vi "timer_correct_rollover.vi"(9 "Reset":bool, 10 "Loop Rate(uSec)":u64) -> (0 "Actual Loop Rate(uSec)":u64, 1 "Late? (Latched)":bool, 2 "Tick Count(uSec)":u64)   [LabVIEW 2014]
doc: "This VI will monitor the rate of a loop on FPGA. It calculates the number of ticks that have passed since the last call and compares it with the desired count. If more ticks have passed than desired, the Late? Boolean latches to TRUE until reset.\n\n<B>Inputs:</B>\n<B>Count(Ticks)</B> - The desired number of ticks since the last call.\n<B>Reset</B> - Resets the Late? Boolean.\n\n<B>Outputs:</B>\n<B>Tick Count (Ticks)</B> - Returns the value of the free running tick counter.\n<B>Late? (Latched)</B> - Indicates if more FPGA Ticks have passed than the specified number. This Boolean value is latched until reset.\n<B>Actual Loop Rate (Ticks)</B> - The number of ticks that have passed since the last call."
uses:
  Instance           2 36Saved   Monitor Loop Rate - Latching .vi
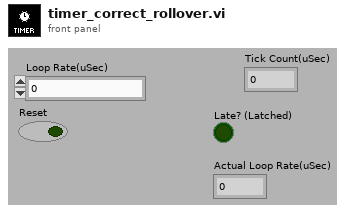
[diagram p1: front panel]
types:
  T1 = cluster{bool, "code":i32, "error_message":string}
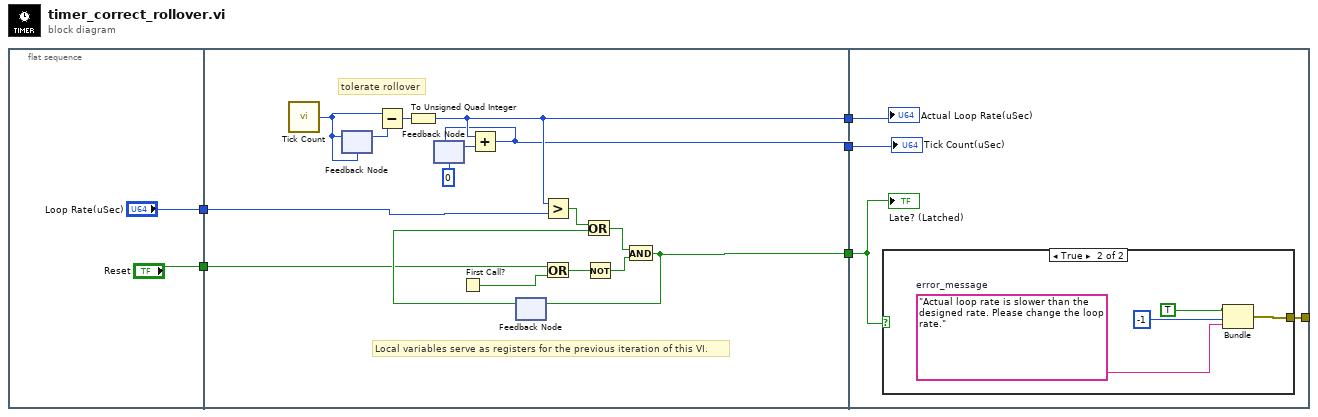
[diagram p0: block diagram]
diagram:
  n1 = flat-sequence {
    tunnel: ["Loop Rate(uSec)"] -> w4
    tunnel: ["Reset"] -> w3
    tunnel: [w12] -> w5
    tunnel: w4 -> [w11]
    tunnel: w3 -> [w10]
    tunnel: [w9] -> w2
    tunnel: [w8] -> w1
    tunnel: w5 -> [w25]
    tunnel: w2 -> [w27]
    tunnel: w1 -> [w26]
    tunnel: [w24] -> _
    frame #0 {
    }
    frame #1 {
      # "tolerate rollover"
      # "Local variables serve as registers for the previous iteration of this VI."
      n2 = call "Tick Count"() -> ("Tick Count(uSec)"=w13:u32)
      n3 = feedback #1(w13) -> (w17:u32)
      n4 = feedback-in #1(w13) -> ()
      n5 = Subtract(x=w13, y=w17) -> (x-y=w14:u32)
      n6 = To Unsigned Quad Integer(1:w14) -> (0:w9:u64)
      n7 = feedback #2(u64 0 ("Tick Count(uSec)")) -> (w15:u64)
      n8 = First Call?() -> (First Call?: T/F=w22:bool)
      n9 = Add(x=w9, y=w15) -> (x+y=w8:u64)
      n10 = feedback-in #2(w8) -> ()
      n11 = feedback #3() -> (w18:bool)  [unwired: 1 in]
      n12 = Greater?(x=w9, y=w11) -> (0:w23:bool)
      n13 = Or(x=w10, y=w22) -> (x .or. y?=w21:bool)
      n14 = Or(x=w23, y=w18) -> (x .or. y?=w20:bool)
      n15 = Not(x=w21) -> (.not. x?=w19:bool)
      n16 = And(x=w20, y=w19) -> (x .and. y?=w12:bool)
      n17 = feedback-in #3(w12) -> ()
    }
    frame #2 {
      n18 = case shown="True" w25 {
        tunnel: [_ w28] -> w24
        frame False {
        }
        frame True {
          w31 = "Actual loop rate is slower than the designed rate. Please change the loop rate."  # error_message
          n19 = Bundle(TRUE, "code"=-1, "error_message"=w31) -> (w28:T1)  [unwired: 1 in]
        }
      }
      "Tick Count(uSec)" <- w26
      "Actual Loop Rate(uSec)" <- w27
      "Late? (Latched)" <- w25
    }
  }
